vi "Installation Complete.vi"() -> ()   [LabVIEW 2024, in "Sift Client.lvlib"]
uses:
  Sift Client.lvlib
panel:
  out "?":string
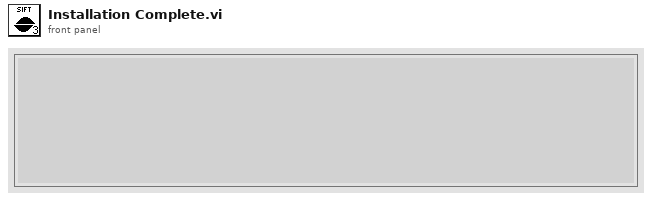
[diagram p1: front panel]
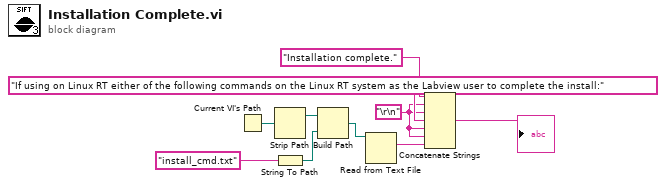
[diagram p0: block diagram]
diagram:
  w3 = "\r\n"
  n1 = Current VI's Path() -> (path=w8:path)
  n2 = Strip Path(path=w8) -> (stripped path=w7:path)  [unwired: 1 out]
  n3 = String To Path(string="install_cmd.txt") -> (path=w9:path)
  n4 = Build Path(base path=w7, name or relative path=w9) -> (appended path=w6:path)
  n5 = Read from Text File(file (use dialog)=w6) -> (text=w1:string)  [unwired: 3 in, 3 out]
  n6 = Concatenate Strings("Installation complete.", w3, w3, "If using on Linux RT either of the following commands on the Linux RT system as the Labview user to complete the install:", w3, w3, w1) -> (→"?":string)
